vi "Estructuras Labview 3.vi"() -> ()   [LabVIEW 2022 SP3]
panel:
  in  "Enum":T1(ring)
  out "Divisi":bool
  out "Multi":bool
  out "Operacion":string
  out "Resta":bool
  out "Suma":bool
  out "Resultado":dbl
  in  "Numeric 2":dbl
  in  "Numeric 1":dbl
  out "Iteraciones":i32
  in  "Stop Button":bool
  # "Se pide diseñar una claculadora de 2 operaciones"
  # "0 : Suma\n1 : Resta\n2 : Multiplicacion\n3 : Division"
  # "COMBO BOX"
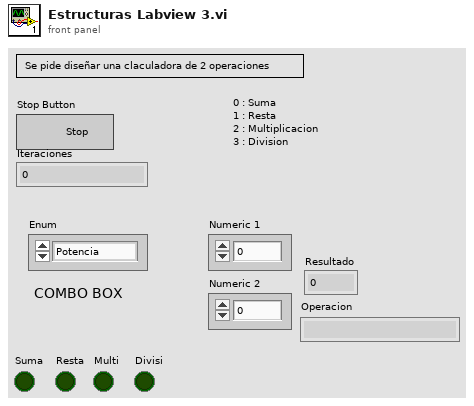
[diagram p1: front panel]
types:
  T1 = enum16{"Potencia", "Suma", "Resta", "Division", "Multiplicacion", ""}
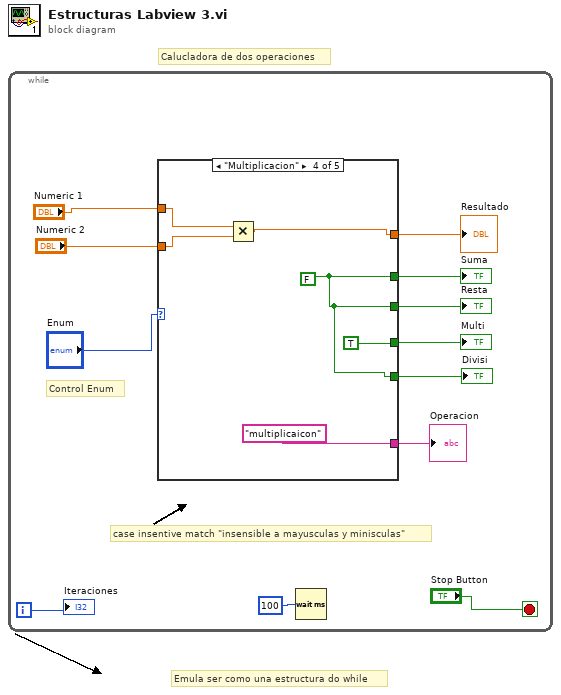
[diagram p0: block diagram]
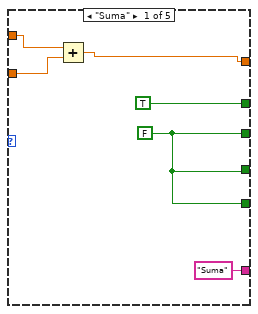
[diagram p2: hidden frame]
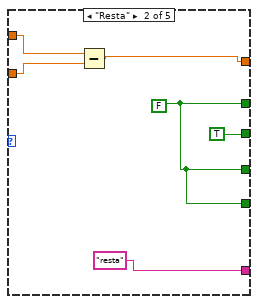
[diagram p3: hidden frame]
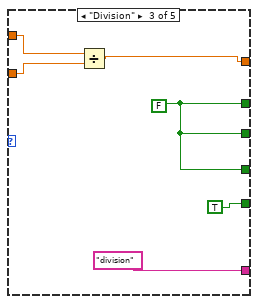
[diagram p4: hidden frame]
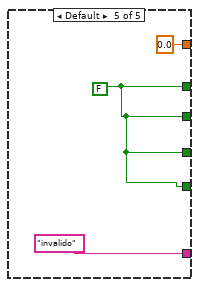
[diagram p5: hidden frame]
diagram:
  # "Emula ser como una estructura do while"
  # "Calucladora de dos operaciones"
  n1 = while {
    i -> [w11]
    stop <- "Stop Button" stop-if-true
    # "Control Enum"
    # "case insentive match \"insensible a mayusculas y minisculas\""
    n2 = case shown="\"Multiplicacion\"" "Enum" {
      tunnel: "Numeric 2" -> [w17 w23 w29 w35 _]
      tunnel: "Numeric 1" -> [w18 w24 w30 w36 _]
      tunnel: [w16 w22 w28 w34 0.0] -> w6
      tunnel: [TRUE w20 w26 w31 w37] -> w5
      tunnel: [w14 TRUE w26 w31 w37] -> w4
      tunnel: [w14 w20 w26 TRUE w37] -> w3
      tunnel: [w14 w20 TRUE w31 w37] -> w2
      tunnel: ["Suma" "resta" "division" "multiplicaicon" "invalido"] -> w1
      frame "Suma" {
        w14 = FALSE
        n3 = Add(x=w18, y=w17) -> (x+y=w16:dbl)
      }
      frame "Resta" {
        w20 = FALSE
        n4 = Subtract(x=w24, y=w23) -> (x-y=w22:dbl)
      }
      frame "Division" {
        w26 = FALSE
        n5 = Divide(x=w30, y=w29) -> (x/y=w28:dbl)
      }
      frame "Multiplicacion" {
        w31 = FALSE
        n6 = Multiply(x=w36, y=w35) -> (x*y=w34:dbl)
      }
      frame Default {
        w37 = FALSE
      }
    }
    "Resultado" <- w6
    "Suma" <- w5
    "Resta" <- w4
    "Operacion" <- w1
    "Multi" <- w3
    "Divisi" <- w2
    n7 = Wait (ms)(milliseconds to wait=u32 100) -> ()  [unwired: 1 out]
    "Iteraciones" <- w11
  }
